vi "CSM - Remove Duplicated Following Messages.vi"(2 "Current State":string, 3 "Remaining States":string) -> (1 "Remaining States Left":string)   [LabVIEW 2017, in "Communicable State Machine.lvlib"]
doc: "### CSM - Remove Duplicated Following Messages.vi\n\n-- <b>Controls</b> --\n- <b>Current State</b>:\n- <b>Remaining States</b>:\n\n-- <b>Indicators</b> --\n- <b>Remaining States Left</b>:"
uses:
  Communicable State Machine.lvlib
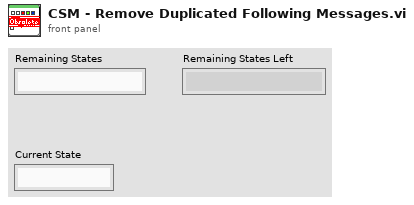
[diagram p1: front panel]
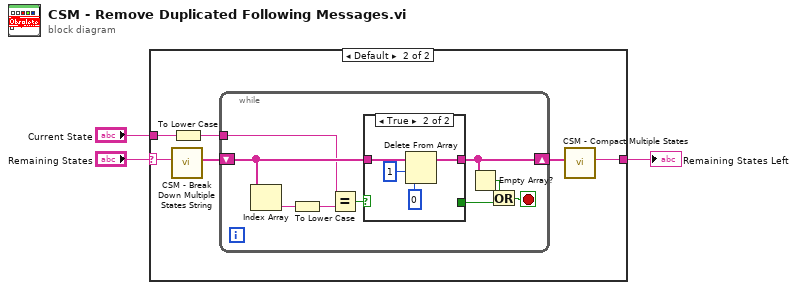
[diagram p0: block diagram]
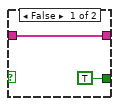
[diagram p3: hidden frame]
diagram:
  n1 = case shown="Default" "Remaining States" {
    selector: "Remaining States" -> [w4 w6]
    tunnel: [w4 w10] -> w3
    tunnel: "Current State" -> [_ w8]
    frame "" {
    }
    frame Default {
      n2 = call "CSM - Break Down Multiple States String.vi"("States"=w6) -> ("Multiple States"=w7:string[])  [unwired: 10 in]
      n3 = To Lower Case(string=w8) -> (all lower case string=w5:string)
      n4 = while {
        tunnel: w5 -> [w17]
        shift-right: [w15] -> w9
        shift-left: w7 -> [w19]
        stop <- w14 stop-if-true
        n5 = Index Array(array=w19) -> (element=w18:string)  [unwired: 1 in]
        n6 = To Lower Case(string=w18) -> (all lower case string=w11:string)
        n7 = Equal?(x=w17, y=w11) -> (x = y?=w16:bool)
        n8 = case shown="True" w16 {
          tunnel: w19 -> [w21 w25]
          tunnel: [w21 w24] -> w15
          tunnel: [TRUE _] -> w13
          frame False {
          }
          frame True {
            n9 = Delete From Array(array=w25, length=1, index=0) -> (array with subset deleted=w24:string[])  [unwired: 1 out]
          }
        }
        n10 = Empty Array?(array=w15) -> (empty?=w12:bool)
        n11 = Or(x=w12, y=w13) -> (x .or. y?=w14:bool)
      }
      n12 = call "CSM - Compact Multiple States.vi"("Multiple States"=w9) -> ("States"=w10:string)  [unwired: 9 in]
    }
  }
  "Remaining States Left" <- w3
